vi "Main.vi"(11 "Module Admin":refnum<class "Delacor_lib_QMH_Module Admin.lvclass">) -> ()   [LabVIEW 2020, in "UI.lvlib"]
doc: "This template is based off of the Queued Message Handler design pattern and the Queued Message Handler project template that ships with LabVIEW.\n\nThe main difference is that the queue is private to this module and communication between modules is performed via Broadcast and Request events.\n\nRequest events are wrapped in public API methods and are handled in the Event Handling Loop (EHL) of this VI. Any module can register for Broadcast events sent by this module. The EHL generates messages based on user interface actions.\n\nThe Message Handling Loop (MHL) processes messages generated by the EHL, or by other messages. The messages are string values, so new messages can be added easily to the Message Cases case structure in the MHL. Each message cluster can also provide an optional value for Message Data, which is a variant that can be converted to whatever message-specific data is required.\n_____\nBased on Delacor QMH Project Template 5.0.0.82."
uses:
  UI.lvlib
  <vilib>/Delacor/Delacor QMH/Libraries/Module Admin_class/Delacor_lib_QMH_Module Admin.lvclass
  Module Data--cluster.ctl
  Stop Argument--cluster.ctl
  <vilib>/Delacor/Delacor QMH/Libraries/Message Queue_class/Delacor_lib_QMH_Message Queue.lvclass/Delacor_lib_QMH_Message Queue.ctl
  <vilib>/Delacor/Delacor QMH/Libraries/Module Admin_class/Delacor_lib_QMH_Module Admin.lvclass/Delacor_lib_QMH_Module Admin.ctl
  <vilib>/Utility/miscctls.llb/LVPointTypeDef.ctl
  <vilib>/Delacor/Delacor QMH/Libraries/Message Queue_class/Delacor_lib_QMH_Enqueue Message (Single).vi
  <vilib>/Delacor/Delacor QMH/Libraries/Module Admin_class/Delacor_lib_QMH_Get External Launch.vi
  <vilib>/Utility/error.llb/Error Cluster From Error Code.vi
  <vilib>/ErrorRing/Error Ring.xnode
  <vilib>/Delacor/Delacor QMH/Libraries/Message Queue_class/Delacor_lib_QMH_Message Queue.lvclass
  Acquisition/Acquisition.lvlib
  Analisis/Analisis.lvlib
  Mensajes/Mensajes.lvlib
  Configuracion/Configuracion.lvlib
  Database/Database.lvlib
panel:
  out "error out":errorcluster
  out "Status":string
  in  "START AQC":bool
  in  "Stop ACQ":bool
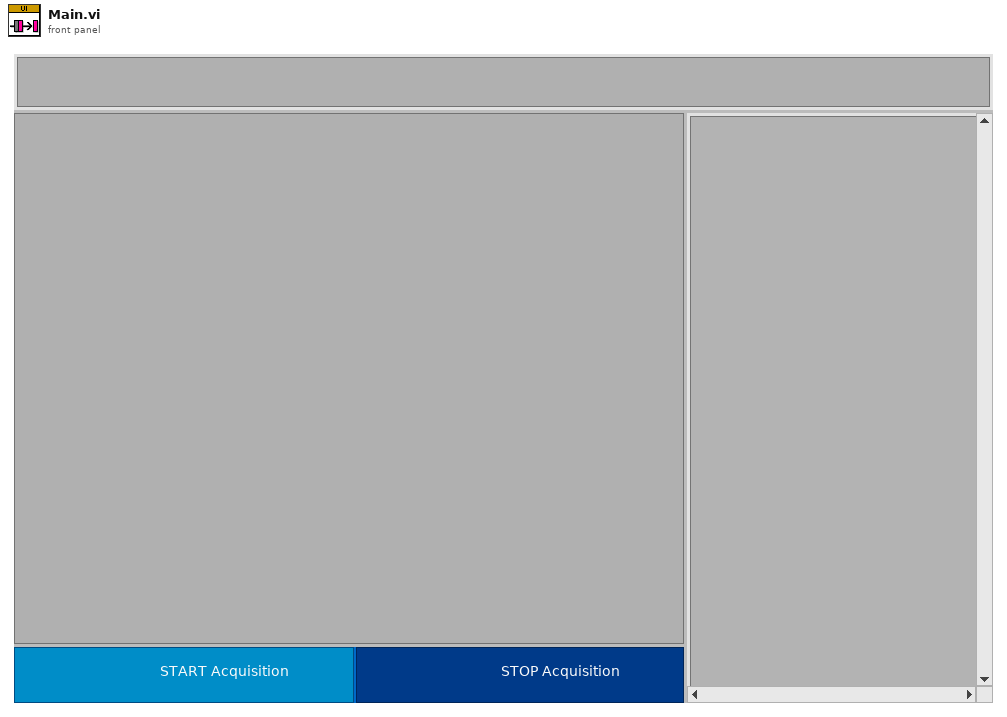
[diagram p1: front panel]
types:
  T1 = typedef "UI.lvlib/Request Events--cluster.ctl" = cluster{"Stop Module":refnum<user-event>, "Show Panel":refnum<user-event>, "Hide Panel":refnum<user-event>, "Get Module Execution Status":refnum<user-event>, "Show Diagram":refnum<user-event>}
  T2 = typedef "Acquisition.lvlib/Broadcast Events--cluster.ctl" = cluster{"Module Did Init":refnum<user-event>, "Status Updated":refnum<user-event>, "Error Reported":refnum<user-event>, "Module Did Stop":refnum<user-event>, "Update Module Execution Status":refnum<user-event>, "Start ACQ":refnum<user-event>}
  T3 = typedef "Analisis.lvlib/Broadcast Events--cluster.ctl" = cluster{"Module Did Init":refnum<user-event>, "Status Updated":refnum<user-event>, "Error Reported":refnum<user-event>, "Module Did Stop":refnum<user-event>, "Update Module Execution Status":refnum<user-event>}
  T4 = typedef "Mensajes.lvlib/Broadcast Events--cluster.ctl" = cluster{"Module Did Init":refnum<user-event>, "Status Updated":refnum<user-event>, "Error Reported":refnum<user-event>, "Module Did Stop":refnum<user-event>, "Update Module Execution Status":refnum<user-event>}
  T5 = typedef "Configuracion.lvlib/Broadcast Events--cluster.ctl" = cluster{"Module Did Init":refnum<user-event>, "Status Updated":refnum<user-event>, "Error Reported":refnum<user-event>, "Module Did Stop":refnum<user-event>, "Update Module Execution Status":refnum<user-event>}
  T6 = typedef "Database.lvlib/Broadcast Events--cluster.ctl" = cluster{"Module Did Init":refnum<user-event>, "Status Updated":refnum<user-event>, "Error Reported":refnum<user-event>, "Module Did Stop":refnum<user-event>, "Update Module Execution Status":refnum<user-event>}
  T7 = typedef "UI.lvlib/Module Data--cluster.ctl" = cluster{"Status":string}
  T8 = enum32{"invalid lock state", "Not Locked", "Locked (No Password)", "Password-protected"}
  T9 = typedef "UI.lvlib/Stop Argument--cluster.ctl" = cluster{"Origin":string, "Exit via Stop Module Req?":bool, "Wait for Module to stop?":bool}
  T10 = enum32{"Invalid", "Standard", "Closed", "Hidden", "Minimized", "Maximized"}
  T11 = typedef "LVPointTypeDef.ctl" = cluster{"Horizontal":i16, "Vertical":i16}
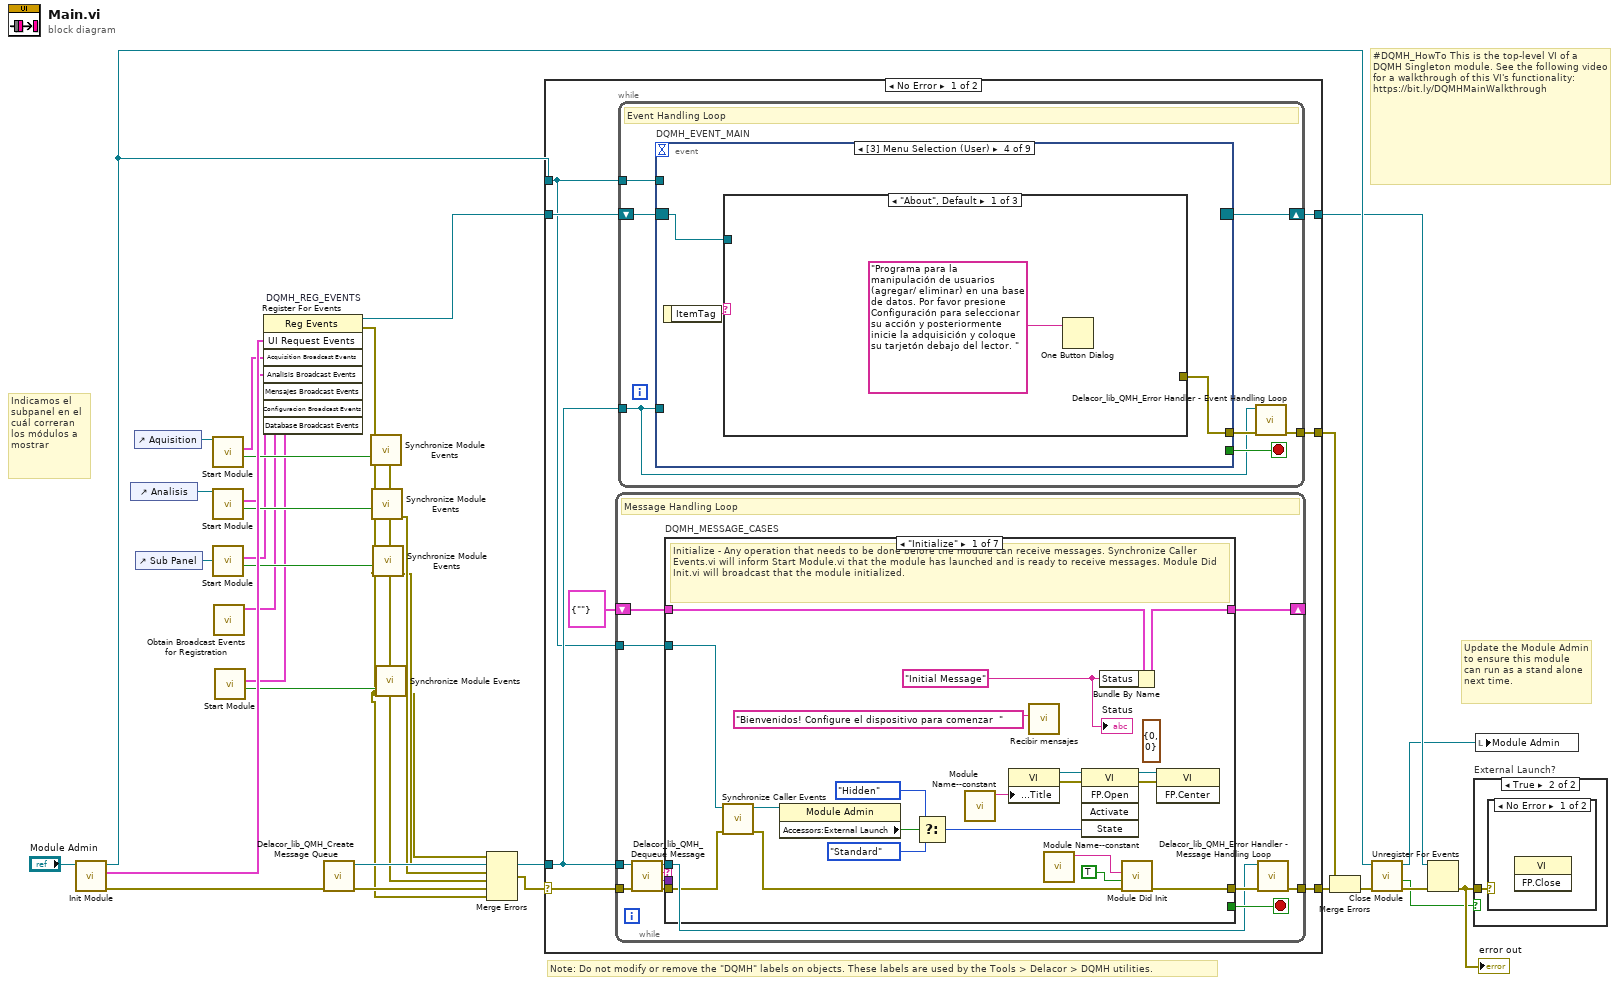
[diagram p0: block diagram]
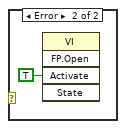
[diagram p3: hidden frame]
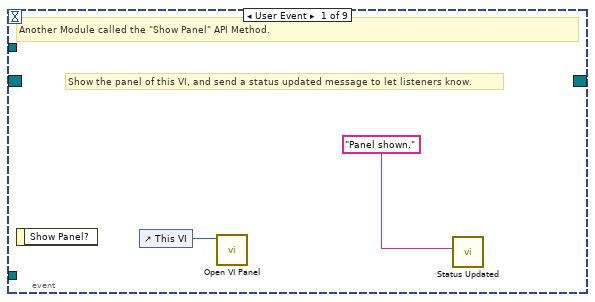
[diagram p4: hidden frame]
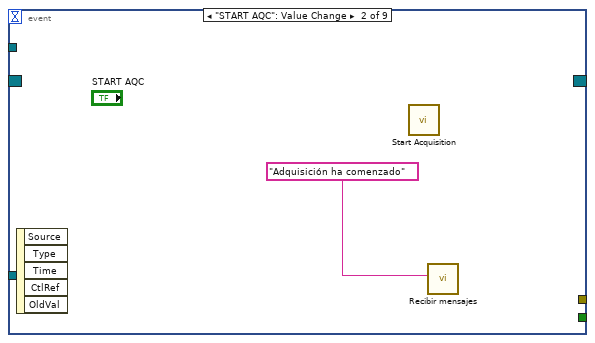
[diagram p5: hidden frame]
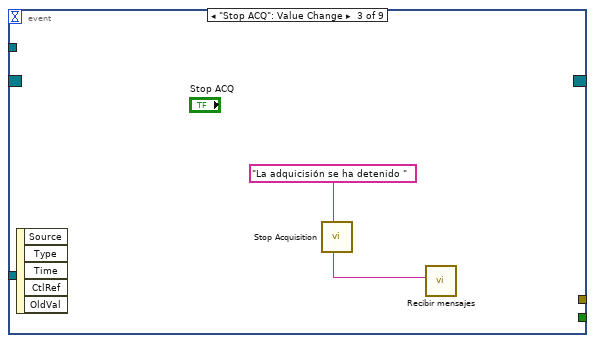
[diagram p6: hidden frame]
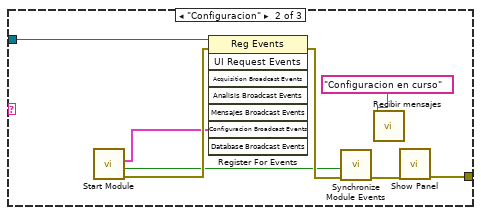
[diagram p7: hidden frame]
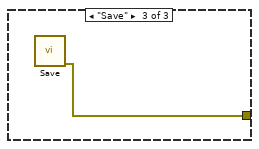
[diagram p8: hidden frame]
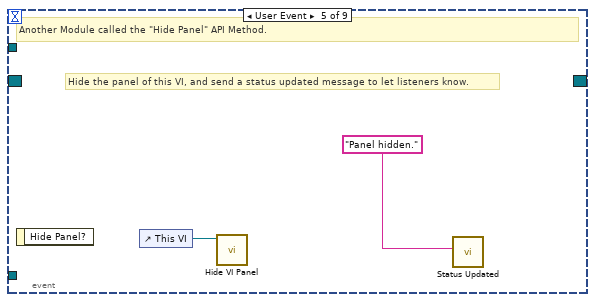
[diagram p9: hidden frame]
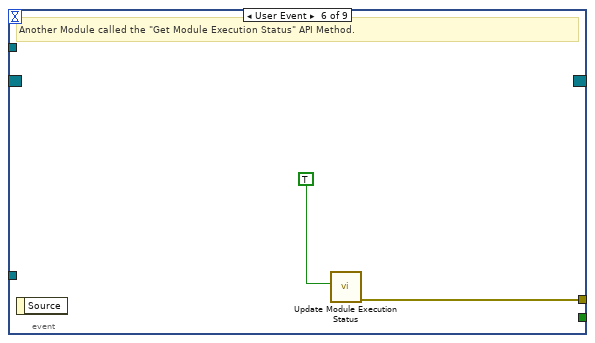
[diagram p10: hidden frame]
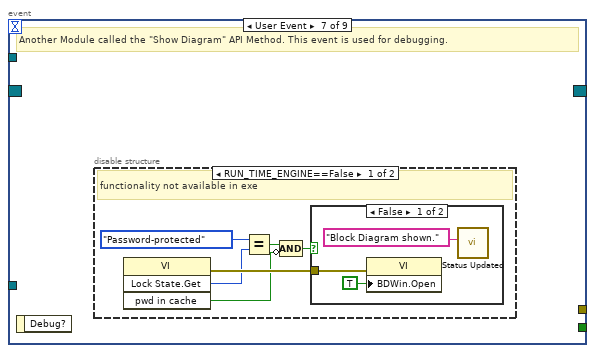
[diagram p11: hidden frame]
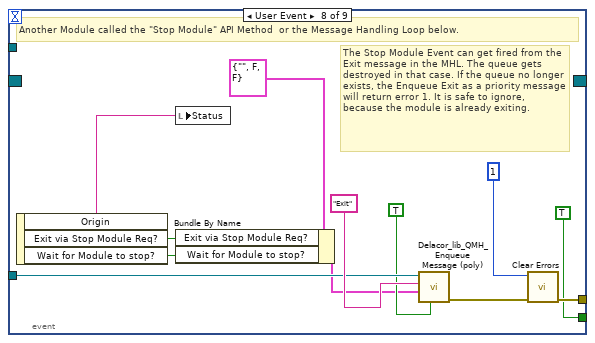
[diagram p14: hidden frame]
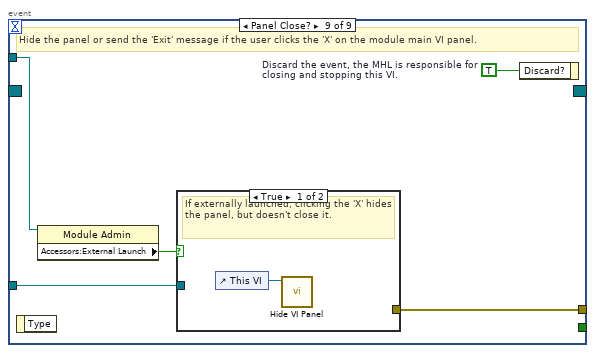
[diagram p15: hidden frame]
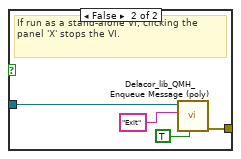
[diagram p16: hidden frame]
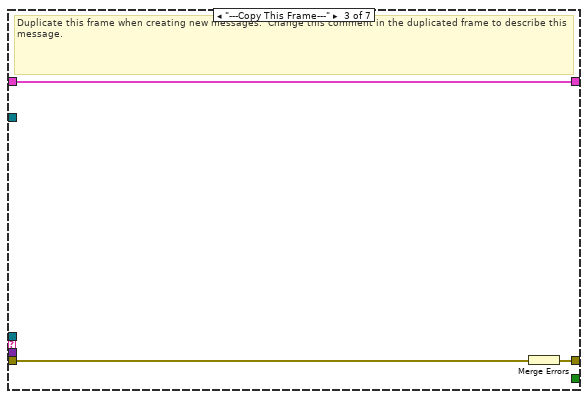
[diagram p18: hidden frame]
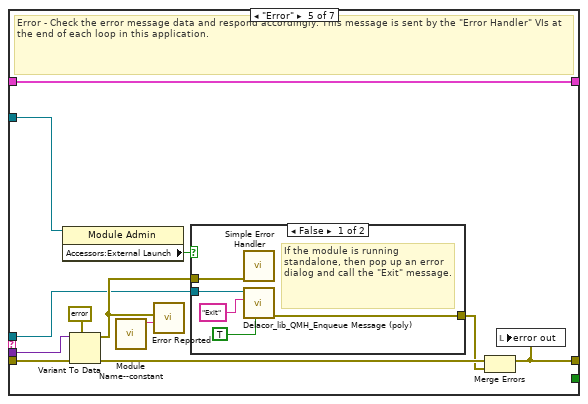
[diagram p20: hidden frame]
diagram:
  # "Indicamos el subpanel en el cuál correran los módulos a mostrar"
  # "#DQMH_HowTo This is the top-level VI of a DQMH Singleton module. See the following video for a walkthrough of this VI's functionality: https://bit.ly/DQMHMainWalkthrough"
  # "Note: Do not modify or remove the \"DQMH\" labels on objects. These labels are used by the Tools > Delacor > DQMH utilities."
  # "Update the Module Admin to ensure this module can run as a stand alone next time."
  n1 = call "Init Module.vi"("Singleton Module Admin in"="Module Admin") -> ("error out"=w32:errorcluster, "UI Request Events"=w22:T1, "Singleton Module Admin out"=w25:refnum<class "Delacor_lib_QMH_Module Admin.lvclass">)  [unwired: 8 in]
  n2 = control-ref of="Analisis"() -> (w1:refnum<vi>)
  n3 = control-ref of="Aquisition"() -> (w3:refnum<vi>)
  n4 = control-ref of="Sub Panel"() -> (w2:refnum<vi>)
  n5 = call "Start Module.vi"("Sub Panel 2"=w3) -> ("Wait for Event Sync?"=w16:bool, "Acquisition Broadcast Events"=w17:T2)  [unwired: 7 in, 2 out]
  n6 = call "Start Module.vi"("Sub Panel"=w1) -> ("Wait for Event Sync?"=w13:bool, "Analisis Broadcast Events"=w14:T3)  [unwired: 7 in, 2 out]
  n7 = call "Start Module.vi"("Sub Panel"=w2) -> ("Wait for Event Sync?"=w10:bool, "Mensajes Broadcast Events"=w11:T4)  [unwired: 7 in, 2 out]
  n8 = call "Obtain Broadcast Events for Registration.vi"() -> ("Configuracion Broadcast Events"=w8:T5)  [unwired: 9 in, 2 out]
  n9 = call "Start Module.vi"() -> ("Wait for Event Sync?"=w7:bool, "Database Broadcast Events"=w6:T6)  [unwired: 8 in, 2 out]
  n10 = register-events "DQMH_REG_EVENTS"(w22, w17, w14, w11, w8, w6) -> (reference out=w23:refnum<event-registration>, error out=w5:errorcluster)  [unwired: 2 in]
  n11 = call <vilib>:"Delacor_lib_QMH_Create Message Queue.vi"("error in (no error)"=w32) -> ("error out"=w27:errorcluster, "Message Queue"=w21:refnum<class "Delacor_lib_QMH_Message Queue.lvclass">)  [unwired: 9 in]
  n12 = call "Synchronize Module Events.vi"("error in (no error)"=w5, "Wait for Event Sync?"=w16) -> ("error out"=w15:errorcluster)  [unwired: 9 in]
  n13 = call "Synchronize Module Events.vi"("error in (no error)"=w5, "Wait for Event Sync?"=w13) -> ("error out"=w12:errorcluster)  [unwired: 9 in]
  n14 = call "Synchronize Module Events.vi"("error in (no error)"=w5, "Wait for Event Sync?"=w10) -> ("error out"=w9:errorcluster)  [unwired: 9 in]
  n15 = call "Synchronize Module Events.vi"("error in (no error)"=w5, "Wait for Event Sync?"=w7) -> ("error out"=w4:errorcluster)  [unwired: 9 in]
  n16 = Merge Errors(w4, w9, w12, w15, w27, w5) -> (w26:errorcluster)
  n17 = case shown="No Error" w26 {
    selector: w26 -> [w39 w188]
    tunnel: [w41 w187] -> w33
    tunnel: [w38 w193] -> w24
    tunnel: w23 -> [w36 w193]
    tunnel: w21 -> [w35 w186]
    tunnel: [w40 _] -> w30
    tunnel: w25 -> [w34 w189]
    frame No Error {
      n18 = while {
        tunnel: w35 -> [w103]
        shift-right: [w107] -> _
        shift-left: T7 {"Status"=""} ("Data Cluster") -> [w108]
        tunnel: w39 -> [w111]
        tunnel: [w109] -> w41
        tunnel: w34 -> [w101]
        stop <- w106 stop-if-true
        # "Message Handling Loop"
        n19 = call-dynamic "Delacor_lib_QMH_Dequeue Message.vi"("error in (no error)"=w111, "Message Queue in"=w103) -> ("error out"=w110:errorcluster, "Message Data"=w104:variant, "Message"=w105:string, "Message Queue out"=w102:refnum<class "Delacor_lib_QMH_Message Queue.lvclass">)  [unwired: 6 in]
        n20 = case "DQMH_MESSAGE_CASES" shown="\"Initialize\"" w105 {
          selector: w105 -> [_ _ _ _ _ _ w173]
          tunnel: w102 -> [_ _ _ _ w143 w165 _]
          tunnel: w110 -> [w130 w134 w137 w139 w150 w171 w175]
          tunnel: [w128 w134 w136 w139 w146 w168 w176] -> w112
          tunnel: w108 -> [w119 w133 w135 w138 w145 w164 w174]
          tunnel: [w118 w133 w135 w138 w145 w164 w174] -> w107
          tunnel: [_ _ _ _ _ w163 _] -> w106
          tunnel: w104 -> [_ _ _ _ w144 w162 _]
          tunnel: w101 -> [w120 _ _ _ w142 w157 _]
          frame "Initialize" {
            (unwired) T11 {"Horizontal"=0, "Vertical"=0} ("Origin")
            w114 = "Initial Message" ("Initial Message")
            # "Initialize - Any operation that needs to be done before the module can receive messages. Synchronize Caller Events.vi will inform Start Module.vi that the module has launched and is ready to receive messages. Module Did Init.vi will broadcast that the module initialized."
            n21 = call "Synchronize Caller Events.vi"("error in (no error)"=w130, "Singleton Module Admin in"=w120) -> ("error out"=w129:errorcluster, "Singleton Module Admin out"=w115:refnum<class "Delacor_lib_QMH_Module Admin.lvclass">)  [unwired: 8 in]
            n22 = property class="Module Admin"(reference=w115) -> ("Accessors:External Launch"=w124:bool)  [unwired: 1 in, 2 out]
            n23 = Select(t=T10."Hidden" ("State"), s=w124, f=T10."Standard" ("State")) -> (s? t:f=w121:T10)
            n24 = call "Module Name--constant.vi"() -> ("Module Name"=w127:string)  [unwired: 11 in]
            n25 = property class="VI"("Front Panel.Title"=w127) -> (reference out=w126:refnum<vi>, error out=w132:errorcluster)  [unwired: 2 in]
            n26 = call "Recibir mensajes.vi"("Mensajes"="Bienvenidos! Configure el dispositivo para comenzar  ") -> ()  [unwired: 10 in, 1 out]
            n27 = call "Module Name--constant.vi"() -> ("Module Name"=w116:string)  [unwired: 11 in]
            n28 = invoke class="VI" method="FP.Open"(reference=w126, error in=w132, "State"=w121) -> (reference out=w125:refnum<vi>, error out=w131:errorcluster)  [unwired: 2 in, 3 out]
            n29 = Bundle By Name(cluster=w119, "Status"=w114) -> (w118:T7)
            n30 = call "Module Did Init.vi"("error in (no error)"=w129, "Initialized?"=TRUE, "Origin"=w116) -> ("error out"=w128:errorcluster)  [unwired: 8 in]
            n31 = invoke class="VI" method="FP.Center"(reference=w125, error in=w131) -> ()  [unwired: 1 in, 3 out]
            "Status" <- w114
          }
          frame "--- Module Specific ---" {
            # "Separator -- The following cases handle messages specific to this Module."
          }
          frame "---Copy This Frame---" {
            # "Duplicate this frame when creating new messages.  Change this comment in the duplicated frame to describe this message."
            n32 = Merge Errors(w137) -> (w136:errorcluster)
          }
          frame "--- Exit and Error Handling---" {
            # "Separator - The following cases handle errors and exit messages."
          }
          frame "Error" {
            # "Error - Check the error message data and respond accordingly. This message is sent by the \"Error Handler\" VIs at the end of each loop in this application."
            n33 = property class="Module Admin"(reference=w142) -> ("Accessors:External Launch"=w141:bool)  [unwired: 1 in, 2 out]
            n34 = Variant To Data(error in=w150, type=errorcluster {"status"=FALSE, "code"=0, "source"=""} ("error constant"), Variant=w144) -> (data=w151:errorcluster, error out=w148:errorcluster)
            n35 = call "Module Name--constant.vi"() -> ("Module Name"=w140:string)  [unwired: 11 in]
            n36 = call "Error Reported.vi"("Additional Information"=w140, "Error"=w151) -> ()  [unwired: 9 in, 1 out]
            n37 = case shown="False" w141 {
              tunnel: [w156 _] -> w147
              tunnel: w143 -> [w154 _]
              tunnel: w151 -> [w155 _]
              frame False {
                # "If the module is running standalone, then pop up an error dialog and call the \"Exit\" message."
                n38 = call <vilib>:"Simple Error Handler.vi"("error in (no error)"=w155) -> ()  [unwired: 4 in, 5 out]
                n39 = call-poly <vilib>:"Delacor_lib_QMH_Enqueue Message (poly).vi"("Priority Message? (F)"=TRUE, "Message"="Exit", "Message Queue in"=w154) -> ("error out"=w156:errorcluster)  [unwired: 7 in, 1 out]
              }
              frame True {
                # "If the module was launched externally, calling the Error Reported broadcast VI is the only action performed by the \"Error\" message. The module's caller can then process the error appropriately."
              }
            }
            n40 = Merge Errors(w148, w147) -> (w146:errorcluster)
            n41 = local write "error out"(w146) -> ()
          }
          frame "Exit" {
            w161 = 91  # 91: not all Exit messages will have an argument
            w163 = TRUE  # Stop the VI
            # "Release the message queue reference"
            # "#CodeNeeded - Add any required cleanup code here"
            # "Exit - Exit the application."
            n42 = Variant To Data(error in=w171, type=T9 {"Origin"="", "Exit via Stop Module Req?"=FALSE, "Wait for Module to stop?"=FALSE} ("Stop Argument"), Variant=w162) -> (data=w159:T9, error out=w167:errorcluster)
            n43 = call <vilib>:"Clear Errors.vi"("error in (no error)"=w167, "specific error code to clear (0: all)"=w161) -> ("error out"=w170:errorcluster)  [unwired: 4 in, 1 out]
            n44 = control-ref of="This VI"() -> (w158:refnum<vi>)
            n45 = call-dynamic "Delacor_lib_QMH_Release Message Queue.vi"("error in (no error)"=w170, "Message Queue"=w165) -> ("error out"=w169:errorcluster)  [unwired: 9 in]
            n46 = call "Handle Exit.vi"("Stop Argument"=w159, "Admin in"=w157, "VI reference"=w158) -> ("error out"=w166:errorcluster)  [unwired: 7 in, 1 out]
            n47 = Merge Errors(w169, w166) -> (w168:errorcluster)
            n48 = call "Stop Module.vi"() -> ()  [unwired: 11 in, 1 out]
            n49 = call "Stop Module.vi"() -> ()  [unwired: 11 in, 1 out]
            n50 = call "Stop Module.vi"() -> ()  [unwired: 11 in, 1 out]
            n51 = call "Stop Module.vi"() -> ()  [unwired: 11 in, 1 out]
          }
          frame Default {
            # "'Default' case only runs if there is a message that isn't defined in any of the other cases.  Output a programming error."
            n52 = call "Module Name--constant.vi"() -> ("Module Name"=w172:string)  [unwired: 11 in]
            n53 = xnode "Error Ring"("parameter 0"=w173, "parameter 1"=w172) -> ("error out"=w177:errorcluster)
            n54 = Merge Errors(w175, w177) -> (w176:errorcluster)
          }
        }
        n55 = call-dynamic "Delacor_lib_QMH_Error Handler - Message Handling Loop.vi"("error in (no error)"=w112, "Message Queue in"=w102) -> ("dup error in"=w109:errorcluster)  [unwired: 8 in, 1 out]
      }
      n56 = while {
        tunnel: w35 -> [w42]
        shift-right: [w45] -> w38
        shift-left: w36 -> [w46]
        tunnel: [w47] -> w40
        tunnel: w34 -> [w43]
        stop <- w44 stop-if-true
        # "Event Handling Loop"
        n57 = event "DQMH_EVENT_MAIN" shown="[3] Menu Selection (User)" {
          selector: w46 -> [_ _ _ w54 _ _ _ _ _]
          dyn-events: [_ _ _ _ _ _ _ _ _] -> w45
          timeout: _ -> [_ _ _ _ _ _ _ _ _]
          tunnel: [_ _ _ _ _ _ _ TRUE ("Discard?") _] -> w44
          tunnel: w42 -> [_ _ _ _ _ _ _ w86 w93]
          tunnel: [_ _ _ w53 _ w69 _ w89 w95] -> w48
          tunnel: w43 -> [_ _ _ _ _ _ _ _ w92]
          event User Event {
            # "Show the panel of this VI, and send a status updated message to let listeners know."
            # "Another Module called the \"Show Panel\" API Method."
            n58 = event-data() -> ()  [unwired: 1 in, 1 out]
            n59 = control-ref of="This VI"() -> (w50:refnum<vi>)
            n60 = call "Open VI Panel.vi"("VI"=w50) -> ()  [unwired: 10 in, 1 out]
            n61 = call "Status Updated.vi"("Status"="Panel shown." ("format string")) -> ()  [unwired: 10 in, 1 out]
          }
          event "START AQC": Value Change {
            n62 = event-data() -> ()  [unwired: 1 in, 5 out]
            n63 = call "Start Acquisition.vi"() -> ()  [unwired: 11 in, 1 out]
            n64 = call "Recibir mensajes.vi"("Mensajes"="Adquisición ha comenzado") -> ()  [unwired: 10 in, 1 out]
          }
          event "Stop ACQ": Value Change {
            n65 = event-data() -> ()  [unwired: 1 in, 5 out]
            n66 = call "Stop Acquisition.vi"() -> ()  [unwired: 11 in, 1 out]
            n67 = call "Recibir mensajes.vi"("Mensajes"="La adquicisión se ha detenido ") -> ()  [unwired: 10 in, 1 out]
          }
          event Menu Selection (User) {
            n68 = event-data() -> ("ItemTag"=w55:string)  [unwired: 1 in]
            n69 = case shown="\"About\", Default" w55 {
              tunnel: w54 -> [_ w64 _]
              tunnel: [_ w62 w65] -> w53
              frame "About", Default {
                n70 = One Button Dialog(message="Programa para la manipulación de usuarios (agregar/ eliminar) en una base de datos. Por favor presione Configuración para seleccionar su acción y posteriormente inicie la adquisición y coloque su tarjetón debajo del lector. ") -> ()  [unwired: 1 in, 1 out]
              }
              frame "Configuracion" {
                n71 = call "Start Module.vi"() -> ("error out"=w61:errorcluster, "Wait for Event Sync?"=w58:bool, "Configuracion Broadcast Events"=w59:T5)  [unwired: 8 in, 1 out]
                n72 = register-events(reference=w64, error in=w61, w59) -> (error out=w60:errorcluster)  [unwired: 5 in, 1 out]
                n73 = call "Synchronize Module Events.vi"("error in (no error)"=w60, "Wait for Event Sync?"=w58) -> ("error out"=w63:errorcluster)  [unwired: 9 in]
                n74 = call "Recibir mensajes.vi"("Mensajes"="Configuracion en curso") -> ()  [unwired: 10 in, 1 out]
                n75 = call "Show Panel.vi"("error in (no error)"=w63) -> ("error out"=w62:errorcluster)  [unwired: 10 in]
              }
              frame "Save" {
                n76 = call "Save.vi"() -> ("error out"=w65:errorcluster)  [unwired: 11 in]
              }
            }
          }
          event User Event {
            # "Hide the panel of this VI, and send a status updated message to let listeners know."
            # "Another Module called the \"Hide Panel\" API Method."
            n77 = event-data() -> ()  [unwired: 1 in, 1 out]
            n78 = control-ref of="This VI"() -> (w67:refnum<vi>)
            n79 = call "Hide VI Panel.vi"("VI"=w67) -> ()  [unwired: 10 in, 1 out]
            n80 = call "Status Updated.vi"("Status"="Panel hidden." ("format string")) -> ()  [unwired: 10 in, 1 out]
          }
          event User Event {
            # "Another Module called the \"Get Module Execution Status\" API Method."
            n81 = event-data() -> ()  [unwired: 1 in, 1 out]
            n82 = call "Update Module Execution Status.vi"("Running?"=TRUE) -> ("error out"=w69:errorcluster)  [unwired: 10 in]
          }
          event User Event {
            # "Another Module called the \"Show Diagram\" API Method. This event is used for debugging."
            n83 = event-data() -> ()  [unwired: 1 in, 1 out]
            n84 = disable-structure shown="RUN_TIME_ENGINE==False" {
              frame condition #0 (active) {
                # "functionality not available in exe"
                n85 = invoke class="VI" method="Lock State.Get"() -> (error out=w75:errorcluster, "Get Lock State"=w74:T8, "pwd in cache"=w71:bool)  [unwired: 4 in, 1 out]
                n86 = Equal?(x=T8."Password-protected", y=w74) -> (x = y?=w72:bool)
                n87 = Compound Arithmetic op=AND(w72, invert w71) -> (w70:bool)
                n88 = case shown="False" w70 {
                  tunnel: w75 -> [w78 _]
                  frame False {
                    n89 = property class="VI"(error in=w78, "BDWin.Open"=TRUE ("Block Diagram Window:Open")) -> ()  [unwired: 1 in, 2 out]
                    n90 = call "Status Updated.vi"("Status"="Block Diagram shown." ("format string")) -> ()  [unwired: 10 in, 1 out]
                  }
                  frame True {
                    # "Password-protected VI, and the password is not in the cache. Do not show the diagram."
                  }
                }
              }
              frame condition #1 {
              }
            }
          }
          event User Event {
            # "The Stop Module Event can get fired from the Exit message in the MHL. The queue gets destroyed in that case. If the queue no longer exists, the Enqueue Exit as a priority message will return error 1. It is safe to ignore, because the module is already exiting."
            # "Another Module called the \"Stop Module\" API Method  or the Message Handling Loop below."
            n91 = event-data() -> ("Origin"=w85:string, "Exit via Stop Module Req?"=w81:bool, "Wait for Module to stop?"=w80:bool)  [unwired: 1 in]
            n92 = local write "Status"(w85) -> ()
            n93 = Bundle By Name(cluster=T9 {"Origin"="", "Exit via Stop Module Req?"=FALSE, "Wait for Module to stop?"=FALSE} ("Stop Argument"), "Exit via Stop Module Req?"=w81, "Wait for Module to stop?"=w80) -> (w79:T9)
            n94 = call-poly <vilib>:"Delacor_lib_QMH_Enqueue Message (poly).vi"("Priority Message? (F)"=TRUE, "Message Data"=w79, "Message"="Exit", "Message Queue in"=w86) -> ("error out"=w90:errorcluster)  [unwired: 6 in, 1 out]
            n95 = call <vilib>:"Clear Errors.vi"("error in (no error)"=w90, "specific error code to clear (0: all)"=1) -> ("error out"=w89:errorcluster)  [unwired: 4 in, 1 out]
          }
          event Panel Close? {
            w94 = TRUE  # Discard the event, the MHL is responsible for closing and stopping this VI.
            # "Hide the panel or send the 'Exit' message if the user clicks the 'X' on the module main VI panel."
            n96 = event-data() -> ()  [unwired: 1 in, 1 out]
            n97 = property class="Module Admin"(reference=w92) -> ("Accessors:External Launch"=w91:bool)  [unwired: 1 in, 2 out]
            n98 = case shown="True" w91 {
              tunnel: w93 -> [_ w99]
              tunnel: [_ w100] -> w95
              frame True {
                # "If externally launched, clicking the 'X' hides the panel, but doesn't close it."
                n99 = control-ref of="This VI"() -> (w96:refnum<vi>)
                n100 = call "Hide VI Panel.vi"("VI"=w96) -> ()  [unwired: 10 in, 1 out]
              }
              frame False {
                # "If run as a stand-alone VI, clicking the panel 'X' stops the VI."
                n101 = call-poly <vilib>:"Delacor_lib_QMH_Enqueue Message (poly).vi"("Priority Message? (F)"=TRUE, "Message"="Exit", "Message Queue in"=w99) -> ("error out"=w100:errorcluster)  [unwired: 7 in, 1 out]
              }
            }
            n102 = event-data("Discard?"=w94) -> ()  [unwired: 1 in, 1 out]
          }
        }
        n103 = call-dynamic "Delacor_lib_QMH_Error Handler - Event Handling Loop.vi"("error in (no error)"=w48, "Message Queue in"=w42) -> ("dup error in"=w47:errorcluster)  [unwired: 8 in, 1 out]
      }
    }
    frame Error {
      # "Synchronize Caller Events.vi will inform Start Module.vi that the module has launched and will let the code calling Start Module.vi register for broadcasts and would permit the caller receive the broadcast that an error occurred at launch time."
      n104 = call-dynamic "Delacor_lib_QMH_Release Message Queue.vi"("error in (no error)"=w188, "Message Queue"=w186) -> ("error out"=w187:errorcluster)  [unwired: 9 in]
      n105 = call "Synchronize Caller Events.vi"("Singleton Module Admin in"=w189) -> ("error out"=w194:errorcluster)  [unwired: 9 in, 1 out]
      n106 = call "Module Name--constant.vi"() -> ("Module Name"=w192:string)  [unwired: 11 in]
      n107 = Format Into String(format string="An error occurred during initialization. %s is no longer running.", w192) -> (resulting string=w190:string)  [unwired: 2 in, 1 out]
      n108 = Merge Errors(w187, w194) -> (w195:errorcluster)
      n109 = call "Error Reported.vi"("Additional Information"=w190, "Error"=w195) -> ()  [unwired: 9 in, 1 out]
    }
  }
  n110 = Merge Errors(w30, w33) -> (w29:errorcluster)
  n111 = call "Close Module.vi"("error in (no error)"=w29, "Module Admin in"=w25) -> ("error out"=w31:errorcluster, "External Launch"=w18:bool, "Module Admin out"=w19:refnum<class "Delacor_lib_QMH_Module Admin.lvclass">)  [unwired: 7 in]
  n112 = Unregister For Events(event registration refnum=w24, error in=w31) -> (error out=w28:errorcluster)
  "error out" <- w28
  n113 = case "External Launch?" shown="True" w18 {
    tunnel: w28 -> [_ w196]
    frame False {
    }
    frame True {
      n114 = case shown="No Error" w196 {
        frame No Error {
          n115 = invoke class="VI" method="FP.Close"() -> ()  [unwired: 3 in, 3 out]
        }
        frame Error {
          n116 = invoke class="VI" method="FP.Open"("Activate"=TRUE ("Activate?")) -> ()  [unwired: 4 in, 5 out]
        }
      }
    }
  }
  n117 = local write "Module Admin"(w19) -> ()
